vi "Insert.vi"(8 "error in":errorcluster caption="错误输入（无错误）", 10 "Data":variant, 11 "PanelRootNode 输入":refnum<class "PanelRootNode.lvclass"> caption="DNL_LabVIEW Object in") -> (0 "error out":errorcluster caption="错误输出", 3 "PanelRootNode 输出":refnum<class "PanelRootNode.lvclass"> caption="DNL_LabVIEW Object out")   [LabVIEW 2013, in "PanelRootNode.lvclass"]
uses:
  PanelRootNode.lvclass
  PanelObject/PanelObject.lvclass
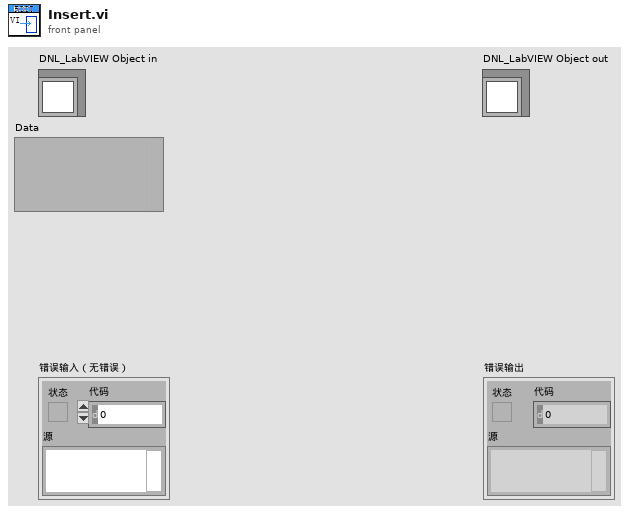
[diagram p1: front panel]
types:
  T1 = cluster{"Node*":refnum<data-value>, "VI*":refnum<vi>}
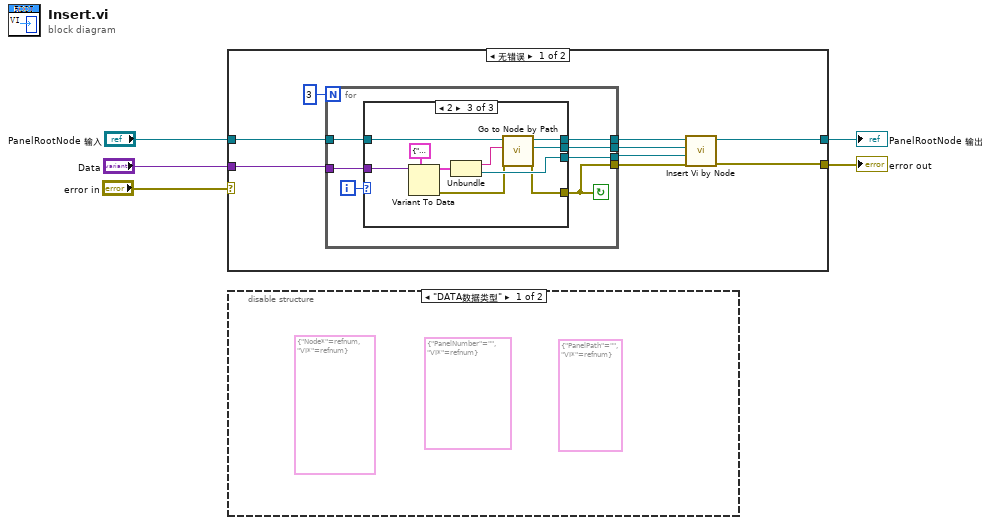
[diagram p0: block diagram]
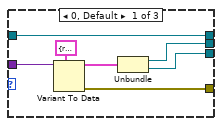
[diagram p3: hidden frame]
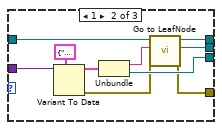
[diagram p4: hidden frame]
diagram:
  n1 = case shown="无错误" "error in" {
    selector: "error in" -> [_ w50]
    tunnel: [w7 w50] -> w4
    tunnel: [w8 w49] -> w2
    tunnel: "PanelRootNode 输入" -> [w14 w49]
    tunnel: "Data" -> [w6 _]
    frame No Error {
      n2 = for {
        N: 3 -> [_]
        tunnel: [w20] -> w10
        tunnel: [w19] -> w12
        tunnel: w14 -> [w18]
        tunnel: [w17] -> w11
        tunnel: [w16] -> w9
        tunnel: w6 -> [w15]
        i -> [w21]
        stop <- w16 continue-if-true
        n3 = case shown="2" w21 {
          tunnel: [w28 w38 w48] -> w17
          tunnel: [w27 w34 w44] -> w19
          tunnel: [w24 w36 w46] -> w20
          tunnel: [w25 w33 w43] -> w16
          tunnel: w18 -> [w24 w31 w42]
          tunnel: w15 -> [w23 w30 w40]
          frame 0, Default {
            n4 = Variant To Data(type=T1 {"Node*"=refnum, "VI*"=refnum}, Variant=w23) -> (data=w26:T1, error out=w25:errorcluster)  [unwired: 1 in]
            n5 = Unbundle(w26) -> ("Node*"=w27:refnum<data-value>, "VI*"=w28:refnum<vi>)
          }
          frame 1 {
            n6 = Variant To Data(type=cluster{"PanelNumber":string, "VI*":refnum<vi>} {"PanelNumber"="", "VI*"=refnum}, Variant=w30) -> (data=w37:cluster{"PanelNumber":string, "VI*":refnum<vi>}, error out=w32:errorcluster)  [unwired: 1 in]
            n7 = Unbundle(w37) -> ("PanelNumber"=w35:string, "VI*"=w38:refnum<vi>)
            n8 = call-dynamic "Go to LeafNode.vi"("error in"=w32, "LeafNumber"=w35, "PanelRootNode 输入"=w31) -> ("error out"=w33:errorcluster, "Node*"=w34:refnum<data-value>, "PanelRootNode 输出"=w36:refnum<class "PanelRootNode.lvclass">)  [unwired: 5 in, 1 out]
          }
          frame 2 {
            n9 = Variant To Data(type=cluster{"PanelPath":string, "VI*":refnum<vi>} {"PanelPath"="", "VI*"=refnum}, Variant=w40) -> (data=w47:cluster{"PanelPath":string, "VI*":refnum<vi>}, error out=w41:errorcluster)  [unwired: 1 in]
            n10 = Unbundle(w47) -> ("PanelPath"=w45:string, "VI*"=w48:refnum<vi>)
            n11 = call-dynamic "Go to Node by Path.vi"("error in"=w41, "NodePath"=w45, "PanelLinkNode 输入"=w42) -> ("error out"=w43:errorcluster, "Node*"=w44:refnum<data-value>, "PanelLinkNode 输出"=w46:refnum<class "PanelRootNode.lvclass">)  [unwired: 5 in, 1 out]
          }
        }
      }
      n12 = call-dynamic "Insert Vi by Node.vi"("error in"=w9, "dynamic VI*"=w11, "Node*"=w12, "PanelRootNode 输入"=w10) -> ("error out"=w7:errorcluster, "PanelRootNode 输出"=w8:refnum<class "PanelRootNode.lvclass">)  [unwired: 6 in]
    }
    frame Error {
    }
  }
  "error out" <- w4
  "PanelRootNode 输出" <- w2
  n13 = disable-structure shown="\"DATA数据类型\"" {
    frame condition #0 {
      (unwired) cluster{"PanelPath":string, "VI*":refnum<vi>} {"PanelPath"="", "VI*"=refnum}
      (unwired) cluster{"PanelNumber":string, "VI*":refnum<vi>} {"PanelNumber"="", "VI*"=refnum}
      (unwired) T1 {"Node*"=refnum, "VI*"=refnum}
    }
    frame condition #1 (active) {
    }
  }
